vi "EventLog.New(array).vi"(7 "Source (All)":T1, 8 "error in (no error)":errorcluster, 9 "Arguments":variant[](array[variant]), 10 "Message (-)":T2, 11 "Level (Info)":T3=enum."Info") -> (0 "error out":errorcluster, 2 "Translated Msg":string)   [LabVIEW 2016]
uses:
  EventLog.EventLevel.ctl
  Translator/Translator.Message.ctl
  EventLog.EventSource.ctl
  EventLog.EventGui.ctl
  EventLog.Event.ctl
  EventLog.Buffer.Action.ctl
  Global/ApplicationGlobal.vi
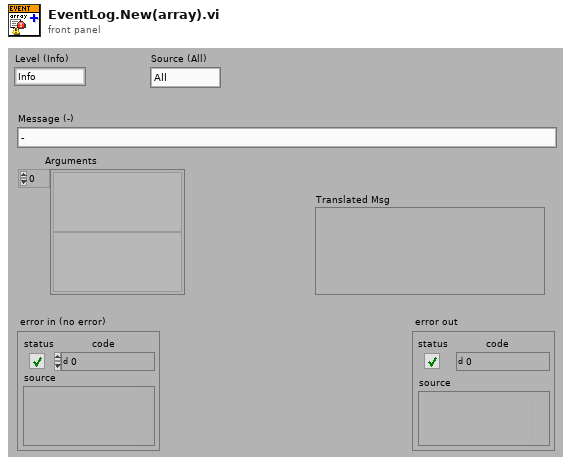
[diagram p1: front panel]
types:
  T1 = typedef "EventLog.EventSource.ctl" = enum16{"All", "Gui", "Cache", "PLC1", "PLC2", "PLC3", "DB", "DB01", "DB02", "DB03", "DB04", "DB05", "DB06", "DB07", "DB08", "DB09", "DB10", "DB11", "DB12", "DB13", "DB14", "DB15", "DB16"}
  T2 = typedef "Translator.Message.ctl" = enum16{"-", "Event confirmed", "Log out", "Log in", "Shutdown", "Cancel", "Start", "Continue", "Stop", "On", "Off", "OK", "NOK", "NOK %s", "This", "Prev", "Home", "Work", "In progress...", "Missing", "Empty", "Hardware failure", "Initial", "Error %d >> %s", "Error %d >> %s >> %s", "Starting %s", "Quitting %s", "Configured", "Initializing", "Quitting", "Loading", "Running %s", "Stopped", "Summary", "Do you want to continue?", "Do you want to exit?", "Log out?", "System", "All", "IDLE", "Translating...%s", "Not found", "Alarm %s", "Run", "Skip", "Abort", "Repeat", "Please wait...", "Database disconnected", "Login to database successful", "Login to database failed: %d; %s", "Get process step data for %s", "Changeover off", "Changeover into %s", "Product %s | %s found in cache with status %d at previous station", "Product %s | %s found in database with status %d at previous station", "Product %s | %s not found in cache at previous station", "Product %s | %s not found in database at previous station", "Product %s | %s found in cache with status %d at this station (%d repetion)", "Product %s | %s found in database with status %d at this station (%d repetition)", "Product %s | %s not found in cache at this station", "Product %s | %s not found in database at this station", "Product %s | %s found in cache for component %s | %s", "Product %s | %s found in database for component %s | %s", "Product not found in cache for component %s | %s", "Product not found in database for component %s | %s", "Product %s | %s connected with component %s | %s (cache)", "Product %s | %s connected with component %s | %s (database)", "New data for %s | %s (cache)", "New data for %s | %s (database)", "File %s moved (cache)", "File %s deleted (cache)", "Msg %d >> %s", "PLC LifeBit Failure", "Reconnecting DB", "Reconnecting PLC", "Free disk space is below 1GB - contact technician", "Unable to check product status", "Product %s SN %s checked in DB"}
  T3 = typedef "EventLog.EventLevel.ctl" = enum8{"Debug", "Info", "Warning", "Error"}
  T4 = typedef "EventLog.Event.ctl" = cluster{"ts":dbl, "lev":T3, "src":T1, "msg":T2, "arg":variant[]}
  T5 = typedef "EventLog.EventGui.ctl" = cluster{"ts":dbl, "lev":T3, "src":T1, "msg":T2, "arg":variant[], "msg_str":string}
  T6 = typedef "EventLog.Buffer.Action.ctl" = enum16{"init", "re-init", "clear", "set translator", "translate", "add", "get"}
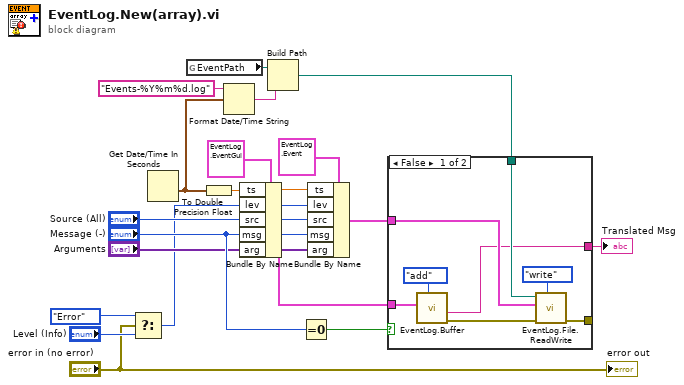
[diagram p0: block diagram]
diagram:
  n1 = Select(t=EventLog.EventLevel."Error", s="error in (no error)", f="Level (Info)") -> (s? t:f=w2:T3)
  n2 = Get Date/Time In Seconds() -> (seconds since 1Jan1904=w10:timestamp)
  n3 = global read "ApplicationGlobal.vi" "EventPath"() -> (w15:path)
  n4 = To Double Precision Float(number=w10) -> (double precision float=w13:dbl)
  n5 = Format Date/Time String(time format string (%c)="Events-%Y%m%d.log", seconds (now)=w10) -> (date/time string=w14:string)  [unwired: 1 in]
  n6 = Bundle By Name(cluster=T5 {"ts"=0.0, "lev"=enum."Debug", "src"=enum."All", "msg"=enum."Log out", "arg"=[], "msg_str"=""} ("Event in"), "ts"=w13, "lev"=w2, "src"="Source (All)", "msg"="Message (-)", "arg"="Arguments") -> (w7:T5)
  n7 = Build Path(base path=w15, name or relative path=w14) -> (appended path=w9:path)
  n8 = Equal To 0?(x="Message (-)") -> (x = 0?=w8:bool)
  n9 = Bundle By Name(cluster=T4 {"ts"=0.0, "lev"=enum."Debug", "src"=enum."All", "msg"=enum."Log out", "arg"=[]} ("event in"), "ts"=w13, "lev"=w2, "src"="Source (All)", "msg"="Message (-)", "arg"="Arguments") -> (w17:T4)
  n10 = case shown="False" w8 {
    tunnel: w7 -> [w21 _]
    tunnel: w17 -> [w26 _]
    tunnel: w9 -> [w24 _]
    tunnel: [w23 _] -> _
    tunnel: [w22 _] -> w5
    frame False {
      n11 = call "EventLog.Buffer.vi"("action (get)"=EventLog.Buffer.Action."add" ("action (read)"), "Event in"=w21) -> ("error out"=w20:errorcluster, "Translated Msg"=w22:string)  [unwired: 6 in, 2 out]
      n12 = call "EventLog.File.ReadWrite.vi"("action (read)"=enum16{"read", "write"}."write", "error in"=w20, "event in"=w26, "file"=w24) -> ("error out"=w23:errorcluster)  [unwired: 3 in, 4 out]
    }
    frame True {
    }
  }
  "Translated Msg" <- w5
  "error out" <- "error in (no error)"
